vi "CalculateD.vi"(11 "Cluster In":T1) -> (3 "Cluster Out":T1)   [LabVIEW 2020]
doc: "Calculate distance from specific point to (0,0,0)."
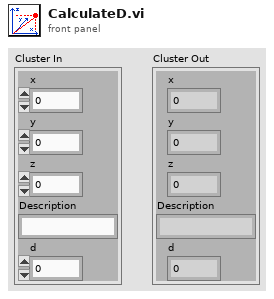
[diagram p1: front panel]
types:
  T1 = cluster{"x":dbl, "y":dbl, "z ":dbl, "Description":string, "d":dbl}
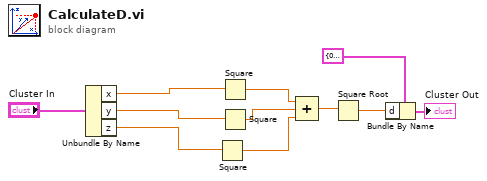
[diagram p0: block diagram]
diagram:
  n1 = Unbundle By Name("Cluster In") -> ("x"=w2:dbl, "y"=w3:dbl, "z"=w4:dbl)
  n2 = Square(x=w4) -> (x^2=w7:dbl)
  n3 = Square(x=w2) -> (x^2=w5:dbl)
  n4 = Square(x=w3) -> (x^2=w6:dbl)
  n5 = Compound Arithmetic op=ADD(w5, w6, w7) -> (w8:dbl)
  n6 = Square Root(x=w8) -> (sqrt(x)=w10:dbl)
  n7 = Bundle By Name(cluster=T1 {"x"=0.0, "y"=0.0, "z "=0.0, "Description"="", "d"=0.0} ("Cluster In 2"), "d"=w10) -> (→"Cluster Out":T1)
